vi "Write InitVal.vi"(8 "error in (no error)":errorcluster, 10 "InitVal":u8, 11 "O3 Generator Power STEP in":refnum<class "O3 Generator Power STEP.lvclass">) -> (0 "error out":errorcluster, 3 "O3 Generator Power STEP out":refnum<class "O3 Generator Power STEP.lvclass">)   [LabVIEW 2014, in "O3 Generator Power STEP.lvclass"]
uses:
  O3 Generator Power STEP.lvclass
  O3 Generator Power STEP.lvclass/O3 Generator Power STEP.ctl
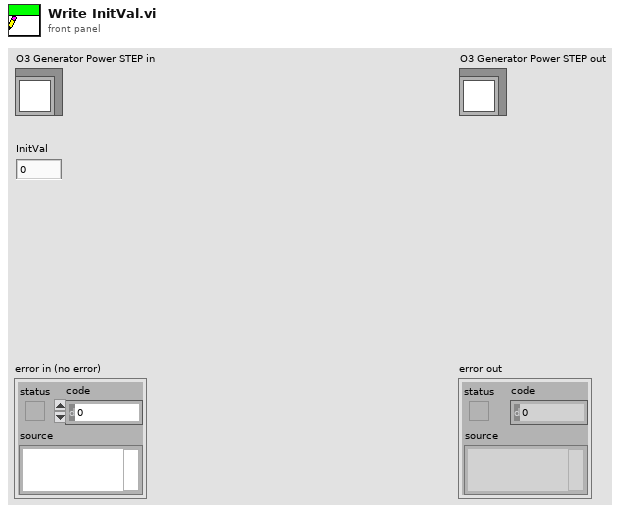
[diagram p1: front panel]
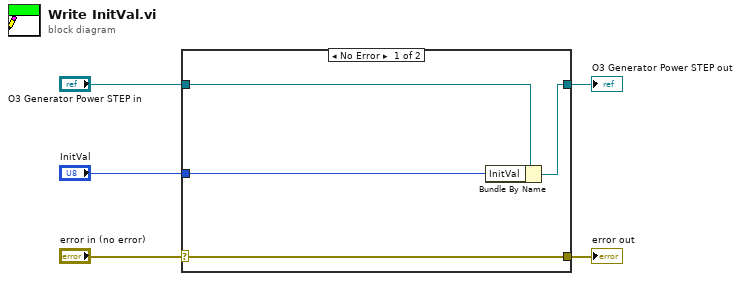
[diagram p0: block diagram]
diagram:
  n1 = case shown="No Error" "error in (no error)" {
    selector: "error in (no error)" -> [w9 w10]
    tunnel: [w9 w10] -> w4
    tunnel: [w7 w11] -> w2
    tunnel: "O3 Generator Power STEP in" -> [w8 w11]
    tunnel: "InitVal" -> [w6 _]
    frame No Error {
      n2 = Bundle By Name(cluster=w8, "InitVal"=w6) -> (w7:refnum<class "O3 Generator Power STEP.lvclass">)
    }
    frame Error {
    }
  }
  "error out" <- w4
  "O3 Generator Power STEP out" <- w2
